vi "Magna Power Control Panel.vi"() -> ()   [LabVIEW 2012]
uses:
  Global/GPIB Numbers.vi
panel:
  out "Status":string
  out "Positive leads?\n(Right to left)":bool
  out "Interpolated Field (T)":dbl format="%_4g"
  in  "Specify\nCurrent or Field?":bool=TRUE
  in  "Desired Field":dbl format="%.2f"
  in  "Read":bool
  in  "Send to power supply":bool
  in  "On?":bool
  in  "stop":bool
  out "Actual Voltage (V)":string
  out "Actual Current (A)":string
  in  "Time between reads (ms)":i32
  in  "Read Continuously?":bool
  out "error out":errorcluster
  in  "Desired Current":dbl format="%.2f"
  in  "Voltage Limit":dbl=2255.0 format="%.2f"
  in  "error in (no error)":errorcluster
  # "Note: Current/voltage may take 2-3 sec to update\nafter the supply is turned on."
  # "Power Supply Control"
  # "Read from Power Supply"
  # "(Always positive)"
  # "Max = 2255 V"
  # "Max ~ 2.184 A"
  # "Magnetic Field"
  # "A positive field corresponds to a north pole located\non the right when looking straight on at magnet)"
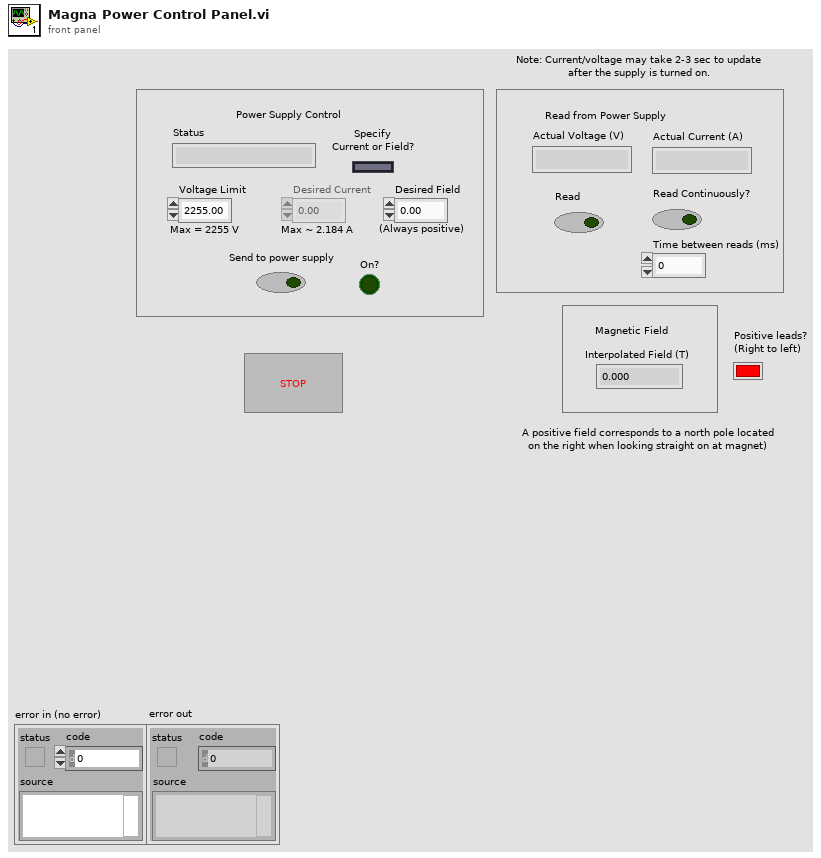
[diagram p1: front panel]
types:
  T1 = cluster{"Name":string, "bus":dbl, "GPIB":dbl, "GPIB as string":string, "byte":i32, "IVI resource name":refnum<k15>, "VISA Resource Name":refnum<visa-resource-name>}
  T2 = cluster{"function (0:volts DC)":u16, "range (0:auto)":u16, "rate (0:slow)":u16, "trigger mode (0:internal)":u16, "Autorange":bool}
  T3 = cluster{"function (0:volts DC)":i16, "range (0:auto)":i16, "rate (0:slow)":i16, "trigger mode (0:internal":i16, "Autorange":bool}
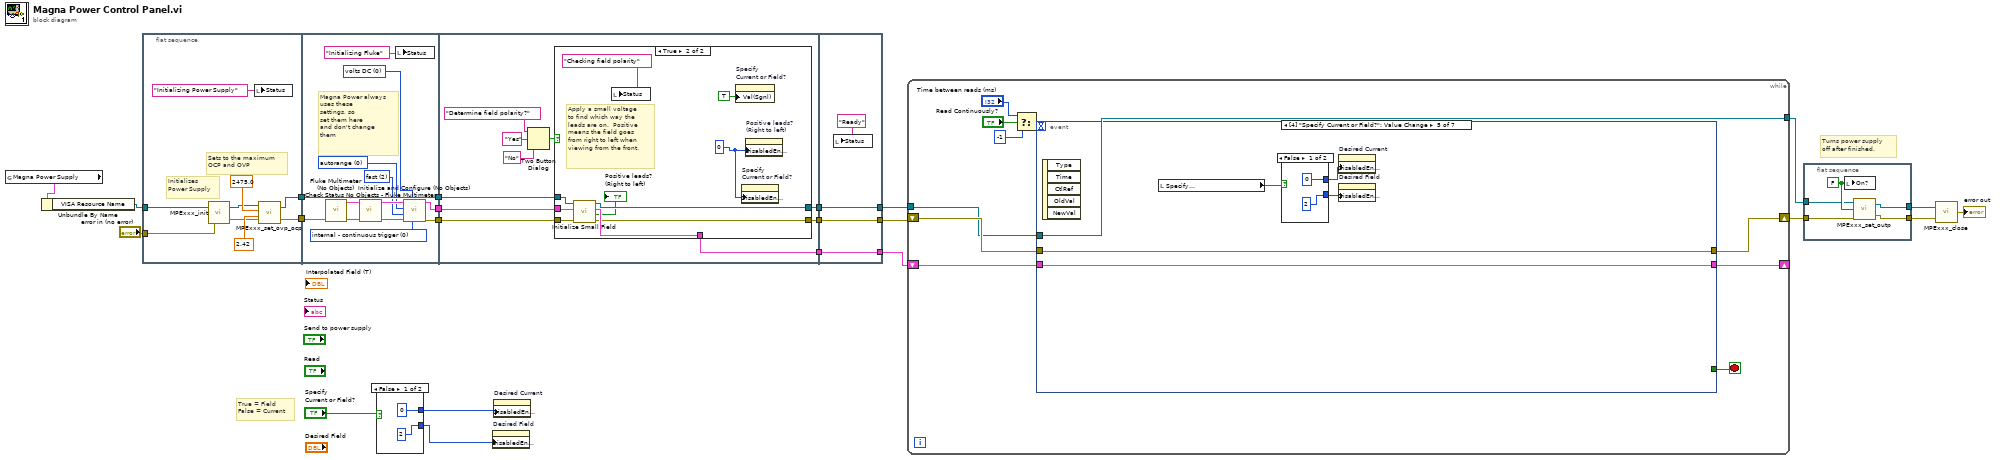
[diagram p0: block diagram]
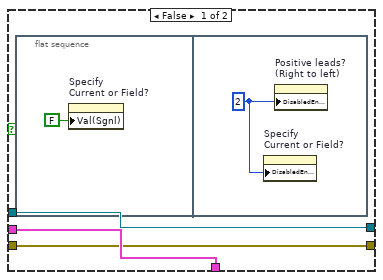
[diagram p2: hidden frame]
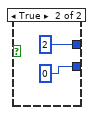
[diagram p3: hidden frame]
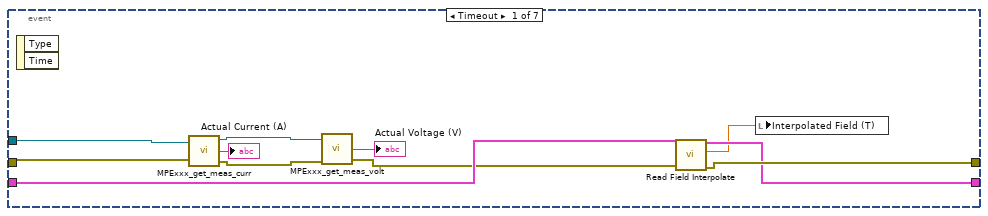
[diagram p4: hidden frame]
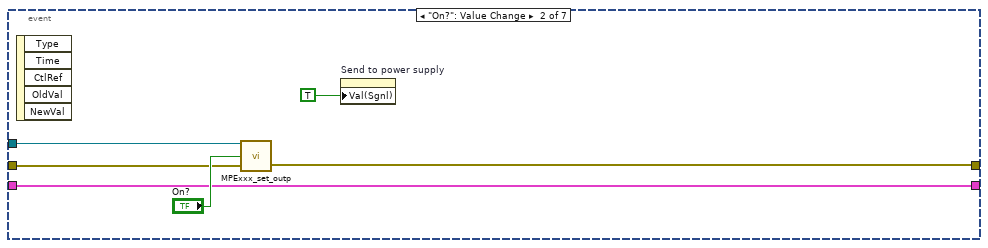
[diagram p5: hidden frame]
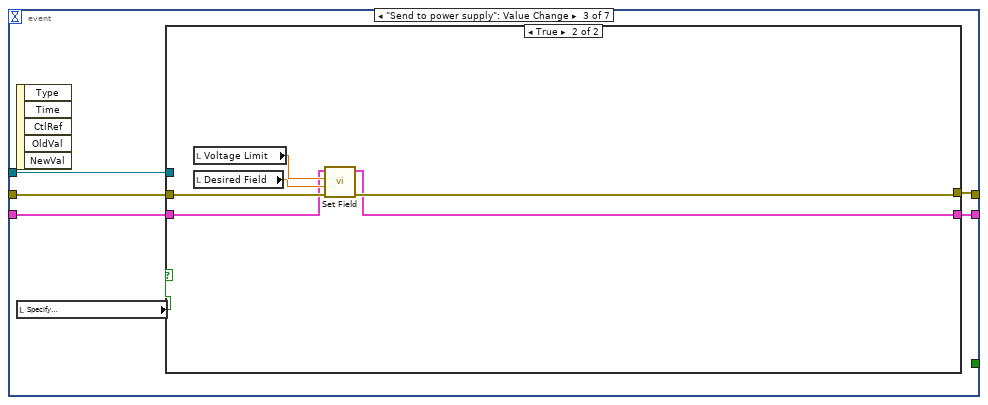
[diagram p6: hidden frame]
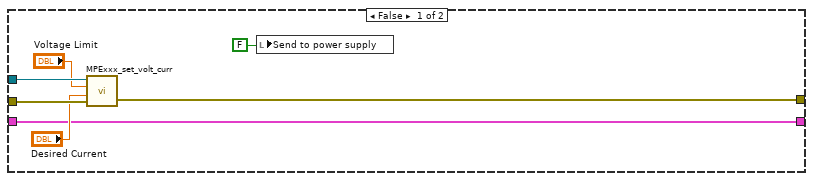
[diagram p7: hidden frame]
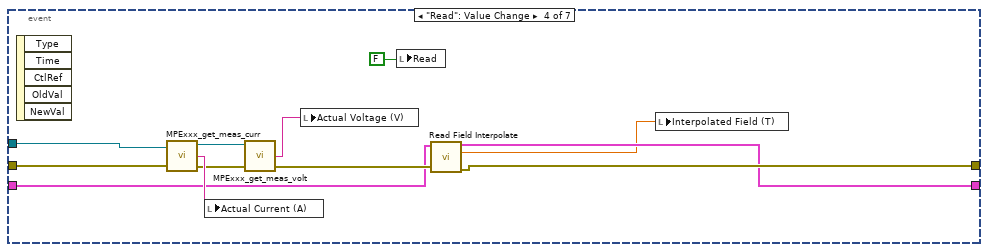
[diagram p8: hidden frame]
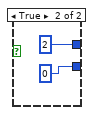
[diagram p9: hidden frame]
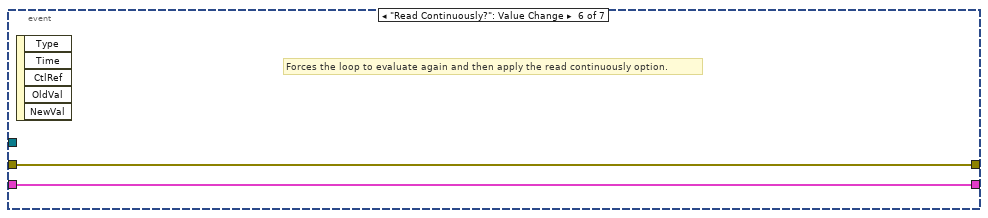
[diagram p10: hidden frame]
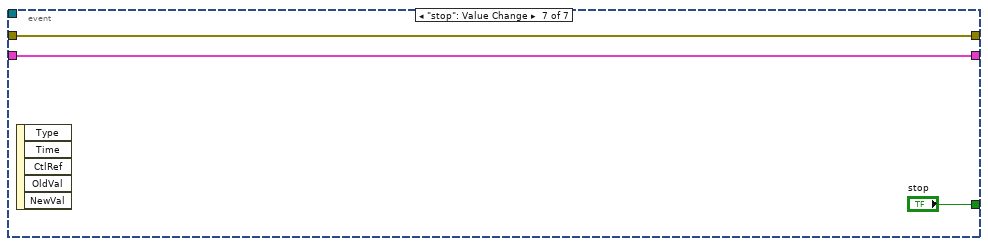
[diagram p11: hidden frame]
diagram:
  # "True = Field\nFalse = Current"
  # "Turns power supply\noff after finished."
  n1 = global read "GPIB Numbers.vi" "Magna Power Supply"() -> (w22:T1)
  n2 = Unbundle By Name(w22) -> ("VISA Resource Name"=w20:refnum<visa-resource-name>)
  n3 = flat-sequence {
    tunnel: "error in (no error)" -> [w29]
    tunnel: w20 -> [w26]
    tunnel: [w25] -> w11
    tunnel: [w24] -> w10
    tunnel: w11 -> [w35]
    tunnel: w10 -> [w44]
    tunnel: [w44] -> w9
    tunnel: [w34] -> w8
    tunnel: [w33] -> w5
    tunnel: w9 -> [w53]
    tunnel: w8 -> [w54]
    tunnel: w5 -> [w49]
    tunnel: [w52] -> w4
    tunnel: [w51] -> w3
    tunnel: [w50] -> w2
    tunnel: [w71] -> w6
    tunnel: [w72] -> w1
    tunnel: [w73] -> w7
    tunnel: w4 -> [w73]
    tunnel: w3 -> [w72]
    tunnel: w2 -> [w71]
    frame #0 {
      # "Initializes\nPower Supply"
      # "Sets to the maximum\nOCP and OVP"
      n4 = call "MPExxx_init.vi"("error in (no error)"=w29, "VISA session"=w26) -> ("error out"=w27:errorcluster, "dup VISA session"=w28:refnum<visa-resource-name>)
      n5 = local write "Status"("Initializing Power Supply" ("Status")) -> ()
      n6 = call "MPExxx_set_ovp_ocp.vi"("error in (no error)"=w27, "Set OCP"=2.42 ("OCP"), "Set OVP"=2475.0 ("OVP"), "VISA session"=w28) -> ("error out"=w25:errorcluster, "dup VISA session"=w24:refnum<visa-resource-name>)
    }
    frame #1 {
      w41 = u16 0 items=["volts DC", "volts AC", "2-wire k.ohms", "4-wire k.ohms", "mA DC", "mA AC"] ("function (0:volts DC)")
      w40 = u16 0 items=["autorange", "200mV, 200 ohms", "2V, 2 kohms", "20V, 20 kohms", "200V, 200 kohms", "1000Vdc, 700 Vac, 2 Mohms", "20 Mohms", "20 mV, 20 ohms"] ("range (0:auto)")
      w39 = u16 2 items=["slow", "medium", "fast"] ("rate (0:slow)")
      w38 = u16 0 items=["internal - continuous trigger", "external - rear panel trigger with delay", "external - bus trigger with delay", "external - rear panel trigger", "external - bus trigger"] ("trigger mode (0:internal)")
      # "Magna Power always\nuses these\nsettings, so\nset them here\nand don't change\nthem"
      n7 = call "Fluke Multimeter (No Objects).vi"("error in (no error)"=w35) -> ("error out"=w36:errorcluster, "Fluke Multimeter out"=w42:T2)  [unwired: 9 in]
      n8 = call "Check Status No Objects - Fluke Multimeter.vi"("error in (no error)"=w36, "input cluster"=w42) -> ("error out"=w37:errorcluster, "output cluster"=w43:T3)  [unwired: 6 in, 2 out]
      n9 = local write "Status"("Initializing Fluke" ("Status")) -> ()
      n10 = call "Initialize and Configure (No Objects).vi"("trigger mode (0:internal)"=w38, "function (0:volts DC)"=w41, "error in (no error)"=w37, "rate (0:slow)"=w39, "range (0:auto)"=w40, "input cluster"=w43) -> ("error out"=w33:errorcluster, "output cluster"=w34:T3)  [unwired: 4 in]
    }
    frame #2 {
      n11 = Two Button Dialog(message="Determine field polarity?", 1:"No" ("F button name (\"Cancel\")"), 2:"Yes" ("T button name (\"OK\")")) -> (T button?=w48:bool)
      n12 = case shown="True" w48 {
        tunnel: w54 -> [w56 w69]
        tunnel: w53 -> [w57 w62]
        tunnel: [w57 w68] -> w52
        tunnel: [w56 w67] -> w51
        tunnel: [w55 w66] -> w50
        tunnel: w49 -> [w55 w65]
        frame False {
          n13 = flat-sequence {
            frame #0 {
              n14 = property on="Specify\nCurrent or Field?" class="Bool (strict)"("Val(Sgnl)"=FALSE ("Value (Signaling)")) -> ()  [unwired: 2 in, 2 out]
            }
            frame #1 {
              w59 = 2
              n15 = property on="Specify\nCurrent or Field?" class="Bool (strict)"("DisabledEnum"=w59) -> ()  [unwired: 2 in, 2 out]
              n16 = property on="Positive leads?\n(Right to left)" class="Bool (strict)"("DisabledEnum"=w59) -> ()  [unwired: 2 in, 2 out]
            }
          }
        }
        frame True {
          w61 = 0
          # "Apply a small voltage\nto find which way the\nleads are on.  Positive\nmeans the field goes\nfrom right to left when\nviewing from the front."
          n17 = call "Initialize Small Field.vi"("error in (no error)"=w65, "input cluster"=w69, "VISA session"=w62) -> ("error out"=w66:errorcluster, "Positive?"=→"Positive leads?\n(Right to left)":bool, "output cluster"=w67:T3, "dup VISA session"=w68:refnum<visa-resource-name>)  [unwired: 5 in]
          n18 = local write "Status"("Checking field polarity" ("Status")) -> ()
          n19 = property on="Specify\nCurrent or Field?" class="Bool (strict)"("Val(Sgnl)"=TRUE ("Value (Signaling)")) -> ()  [unwired: 2 in, 2 out]
          n20 = property on="Specify\nCurrent or Field?" class="Bool (strict)"("DisabledEnum"=w61) -> ()  [unwired: 2 in, 2 out]
          n21 = property on="Positive leads?\n(Right to left)" class="Bool (strict)"("DisabledEnum"=w61) -> ()  [unwired: 2 in, 2 out]
        }
      }
    }
    frame #3 {
      n22 = local write "Status"("Ready" ("Status")) -> ()
    }
  }
  n23 = case shown="False" "Specify\nCurrent or Field?" {
    tunnel: [2 0] -> w12
    tunnel: [0 2] -> w13
    frame False {
    }
    frame True {
    }
  }
  n24 = property on="Desired Field" class="DigNum (strict)"("DisabledEnum"=w12) -> ()  [unwired: 2 in, 2 out]
  n25 = property on="Desired Current" class="DigNum (strict)"("DisabledEnum"=w13) -> ()  [unwired: 2 in, 2 out]
  n26 = while {
    tunnel: w7 -> [w80]
    shift-right: [w81] -> w18
    shift-left: w6 -> [w83]
    tunnel: [w80] -> w15
    shift-right: [w78] -> _
    shift-left: w1 -> [w79]
    stop <- w82 stop-if-true
    n27 = Select(t="Time between reads (ms)", s="Read Continuously?", f=-1) -> (s? t:f=w87:i32)
    n28 = event shown="[4] \"Specify Current or Field?\": Value Change" {
      selector: _ -> [_ _ _ _ _ _ _]
      dyn-events: _ -> [_ _ _ _ _ _ _]
      timeout: w87 -> [_ _ _ _ _ _ _]
      tunnel: w80 -> [w96 w102 w110 w134 _ _ _]
      tunnel: w83 -> [w95 w103 w109 w133 w140 w146 w148]
      tunnel: [_ _ _ _ _ _ "stop"] -> w82
      tunnel: [w92 w101 w108 w128 w140 w146 w148] -> w81
      tunnel: w79 -> [w89 w99 w106 w124 w139 w145 w147]
      tunnel: [w91 w99 w105 w127 w139 w145 w147] -> w78
      event Timeout {
        n29 = event-data() -> ()  [unwired: 1 in, 2 out]
        n30 = call "MPExxx_get_meas_curr.vi"("VISA session"=w96, "error in (no error)"=w95) -> ("dup VISA session"=w93:refnum<visa-resource-name>, "Output Current"=→"Actual Current (A)":string, "error out"=w94:errorcluster)
        n31 = call "MPExxx_get_meas_volt.vi"("VISA session"=w93, "error in (no error)"=w94) -> ("Output Voltage"=→"Actual Voltage (V)":string, "error out"=w88:errorcluster)  [unwired: 1 out]
        n32 = call "Read Field Interpolate.vi"("error in (no error)"=w88, "input cluster"=w89) -> ("error out"=w92:errorcluster, "Field (T)"=w90:dbl, "output cluster"=w91:T3)  [unwired: 7 in]
        n33 = local write "Interpolated Field (T)"(w90) -> ()
      }
      event "On?": Value Change {
        n34 = event-data() -> ()  [unwired: 1 in, 5 out]
        n35 = call "MPExxx_set_outp.vi"("error in (no error)"=w103, "Output Control"="On?", "VISA session"=w102) -> ("error out"=w101:errorcluster)  [unwired: 1 out]
        n36 = property on="Send to power supply" class="Bool (strict)"("Val(Sgnl)"=TRUE) -> ()  [unwired: 2 in, 2 out]
      }
      event "Send to power supply": Value Change {
        n37 = event-data() -> ()  [unwired: 1 in, 5 out]
        n38 = local read "Specify\nCurrent or Field?"() -> (w107:bool)
        n39 = case shown="True" w107 {
          tunnel: w110 -> [w117 _]
          tunnel: w109 -> [w116 w123]
          tunnel: [w115 w122] -> w108
          tunnel: w106 -> [w111 w119]
          tunnel: [w111 w118] -> w105
          frame False {
            n40 = call "MPExxx_set_volt_curr.vi"("error in (no error)"=w116, "Set Current"="Desired Current", "Set Voltage"="Voltage Limit", "VISA session"=w117) -> ("error out"=w115:errorcluster)  [unwired: 1 out]
            n41 = local write "Send to power supply"(FALSE) -> ()
          }
          frame True {
            n42 = local read "Voltage Limit"() -> (w121:dbl)
            n43 = local read "Desired Field"() -> (w120:dbl)
            n44 = call "Set Field.vi"("error in (no error)"=w123, "Desired Field"=w120, "Voltage Limit"=w121, "input cluster"=w119) -> ("error out"=w122:errorcluster, "output cluster"=w118:T3)  [unwired: 6 in]
          }
        }
      }
      event "Read": Value Change {
        n45 = event-data() -> ()  [unwired: 1 in, 5 out]
        n46 = call "MPExxx_get_meas_curr.vi"("VISA session"=w134, "error in (no error)"=w133) -> ("dup VISA session"=w130:refnum<visa-resource-name>, "Output Current"=w132:string, "error out"=w131:errorcluster)
        n47 = local write "Actual Current (A)"(w132) -> ()
        n48 = call "MPExxx_get_meas_volt.vi"("VISA session"=w130, "error in (no error)"=w131) -> ("Output Voltage"=w129:string, "error out"=w125:errorcluster)  [unwired: 1 out]
        n49 = local write "Actual Voltage (V)"(w129) -> ()
        n50 = local write "Read"(FALSE) -> ()
        n51 = call "Read Field Interpolate.vi"("error in (no error)"=w125, "input cluster"=w124) -> ("error out"=w128:errorcluster, "Field (T)"=w126:dbl, "output cluster"=w127:T3)  [unwired: 7 in]
        n52 = local write "Interpolated Field (T)"(w126) -> ()
      }
      event "Specify\nCurrent or Field?": Value Change {
        n53 = event-data() -> ()  [unwired: 1 in, 5 out]
        n54 = local read "Specify\nCurrent or Field?"() -> (w138:bool)
        n55 = case shown="False" w138 {
          tunnel: [2 0] -> w137
          tunnel: [0 2] -> w136
          frame False {
          }
          frame True {
          }
        }
        n56 = property on="Desired Current" class="DigNum (strict)"("DisabledEnum"=w136) -> ()  [unwired: 2 in, 2 out]
        n57 = property on="Desired Field" class="DigNum (strict)"("DisabledEnum"=w137) -> ()  [unwired: 2 in, 2 out]
      }
      event "Read Continuously?": Value Change {
        # "Forces the loop to evaluate again and then apply the read continuously option."
        n58 = event-data() -> ()  [unwired: 1 in, 5 out]
      }
      event "stop": Value Change {
        n59 = event-data() -> ()  [unwired: 1 in, 5 out]
      }
    }
  }
  n60 = flat-sequence {
    tunnel: w18 -> [w153]
    tunnel: [w152] -> w17
    tunnel: [w151] -> w16
    tunnel: w15 -> [w150]
    frame #0 {
      w154 = FALSE
      n61 = local write "On?"(w154) -> ()
      n62 = call "MPExxx_set_outp.vi"("error in (no error)"=w153, "Output Control"=w154, "VISA session"=w150) -> ("error out"=w152:errorcluster, "dup VISA session"=w151:refnum<visa-resource-name>)
    }
  }
  n63 = call "MPExxx_close.vi"("error in (no error)"=w17, "VISA session"=w16) -> ("error out"=→"error out":errorcluster)
